vi "InverseKinematics.vi"(5 "deltaX":dbl, 7 "deltaY":dbl, 8 "L1":dbl, 9 "L0":dbl, 10 "Next Y":dbl, 11 "Next X":dbl) -> (2 "theta1":dbl, 3 "theta0":dbl)   [LabVIEW 2016, in "controllerLibrary.lvlib"]
doc: "This VI uses a mathscript node to perform the Inverse Kinematics, which turns the desired location into a desired joint angle (degrees)."
uses:
  controllerLibrary.lvlib
  <vilib>/imath/engines/lvmath2/RunTimeEngine/ArithmeticOperatorToken/NIMS_ArithmeticOperator_power(S).vi
  <instcachedir>/0/NIMS_ArithmeticOperator_power(S)_1E6AB98FD36540B9B758A69A385A1B47.lvgen/NIMS_ArithmeticOperator_power(S)_1E6AB98FD36540B9B758A69A385A1B47_010.vi
  <vilib>/imath/engines/lvmath2/RunTimeEngine/BuiltInFunctions/acos/NIMS_acos(C).vi
  <instcachedir>/0/NIMS_acos(C)_922B326325C94F82844AE8117C9317D7.lvgen/NIMS_acos(C)_922B326325C94F82844AE8117C9317D7_001.vi
  <vilib>/imathl/engines/lvmath/Functions/Error Handling/Create Error.vi
  <vilib>/imath/engines/lvmath2/RunTimeSupport/NIMS_Complex To Real.vi
  <instcachedir>/0/NIMS_Complex To Real_A9DD49CC305F495FA24B9F5762C73A31.lvgen/NIMS_Complex To Real_A9DD49CC305F495FA24B9F5762C73A31_001.vi
  <vilib>/imath/engines/lvmath2/RunTimeEngine/BuiltInFunctions/rad_to_deg/NIMS_rad_to_deg.vi
  <instcachedir>/0/NIMS_rad_to_deg_A39AFCDDC8C049FCADAAB7FC30B9F5AA.lvgen/NIMS_rad_to_deg_A39AFCDDC8C049FCADAAB7FC30B9F5AA_001.vi
  <vilib>/imath/engines/lvmath2/RunTimeEngine/NodeEndStatement/NIMS_NodeEndStatement_Output.vi
  <instcachedir>/0/NIMS_NodeEndStatement_Output_53EC0D466D134D7ABD903AC30B43404B.lvgen/NIMS_NodeEndStatement_Output_53EC0D466D134D7ABD903AC30B43404B_001.vi
  <vilib>/imath/engines/lvmath2/RunTimeEngine/ErrorHandling/NIMS_Finalize Error.vi
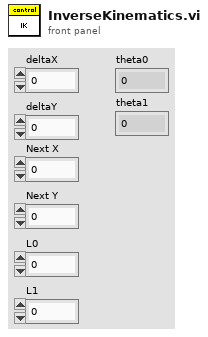
[diagram p1: front panel]
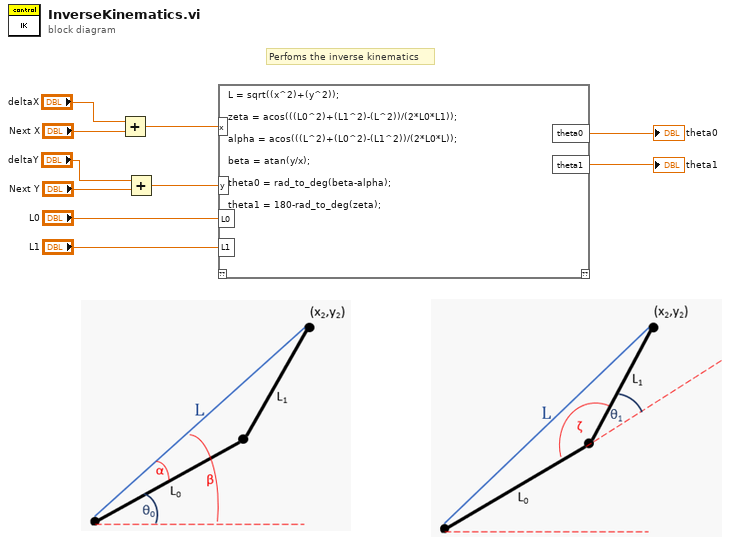
[diagram p0: block diagram]
diagram:
  # "Perfoms the inverse kinematics"
  n1 = Add(x="deltaX", y="Next X") -> (x+y=w4:dbl)
  n2 = Add(x="deltaY", y="Next Y") -> (x+y=w1:dbl)
  n3 = mathscript code="L = sqrt((x^2)+(y^2));\n\nzeta = acos(((L0^2)+(L1^2)-(L^2))/(2*L0*L1));\n\nalpha = acos(((L^2)+(L0^2)-(L1^2))/(2*L0*L));\n\nbeta = atan(y/x);\n\ntheta0 = rad_to_deg(beta-alpha);\n\ntheta1 = 180-rad_to_deg(zeta);"("x"=w4, "y"=w1, "L0"="L0", "L1"="L1") -> ("theta0"=→"theta0":dbl, "theta1"=→"theta1":dbl)  [unwired: 1 in, 1 out]
